vi "fgt get next log.vi"(8 "error in (no error)":errorcluster) -> (0 "error out":errorcluster, 3 "log entry":string)   [LabVIEW 2016, in "fgt_SDK.lvlib"]
doc: "eturns the next log entry stored in memory, if any, and removes it from the queue.\nWill return an error if the queue is empty. Logs are only stored in memory if the corresponding option is set with the fgt_set_log_output_mode function.\nCall this function repeatedly until an error is returned to retrieve all log entries."
uses:
  fgt_SDK.lvlib
  dlls/fgt_SDK_32.dll
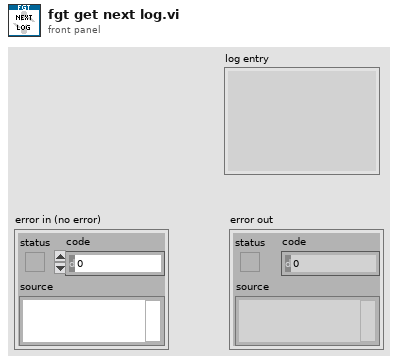
[diagram p1: front panel]
types:
  T1 = typedef "fgt_SDK.lvlib/fgt_STATUS_INFO.ctl" = cluster{"InstrType":T2, "instrSN":u16, "errorCode":u8, "infoCode":u8, "detail":string}
  T2 = typedef "fgt_SDK.lvlib/fgt_INSTRUMENT_TYPE.ctl" = enum32{"None", "MFCS", "MFCS_EZ", "FRP", "LineUP", "IPS", "ESS", "F_OEM", "CFU", "NIFS"}
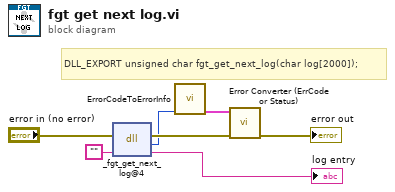
[diagram p0: block diagram]
diagram:
  # "DLL_EXPORT unsigned char fgt_get_next_log(char log[2000]);"
  n1 = dll-call lib="C:/projects/SDK/fgt-sdk-labview/dlls/fgt_SDK_*.*" fn="_fgt_get_next_log@4"(error in="error in (no error)", "log entry"="") -> (error out=w6:errorcluster, "return type"=w4:u8, "log entry"=→"log entry":string)  [unwired: 2 in, 1 out]
  n2 = call "ErrorCodeToErrorInfo.vi"("return type"=w4) -> ("StatusInfo"=w3:T1)  [unwired: 10 in]
  n3 = call "Error Converter (ErrCode or Status).vi"("error in (no error)"=w6, "StatusInfo"=w3) -> ("error out"=→"error out":errorcluster)  [unwired: 9 in]
